vi "Station Detail Main.vi"(8 "error in (no error)":errorcluster, 11 "Vision AI in":refnum<class "Vision AI.lvclass">) -> (0 "error out":errorcluster, 2 "Station Out":T1=enum."ImformOut", 3 "Vision AI out":refnum<class "Vision AI.lvclass">)   [LabVIEW 2019, in "Vision AI.lvclass"]
uses:
  Vision AI.lvclass
  Ctrl/Station Action.ctl
  Ctl/VisionAI Act Step.ctl
  Ctl/S8 PLC to PC Output.ctl
  Ctrl/Auto Inspection Station Name2.ctl
  Ctrl/Auto Inspection Data Name.ctl
  Function/UpVision/Ctrl/UpColorImg.ctl
  <vilib>/userdefined/High Color/IMAQdx.ctl
  Ctl/S8 Station IO.ctl
  Ctrl/ModbusCmd.ctl
  Global/Process Global.vi
  LLB/Commonly VI/Main Glb.vi
  LLB/Commonly VI.lvlib
  Ctrl/MeasureDisplayTab.ctl
  Ctrl/Table Save.ctl
  <vilib>/vision/driver/NI_Vision_Acquisition_Software.lvlib
panel:
  out "CutPath":path[](array[path])
  out "body":string
  out "headers":string
  in  "站別":i32
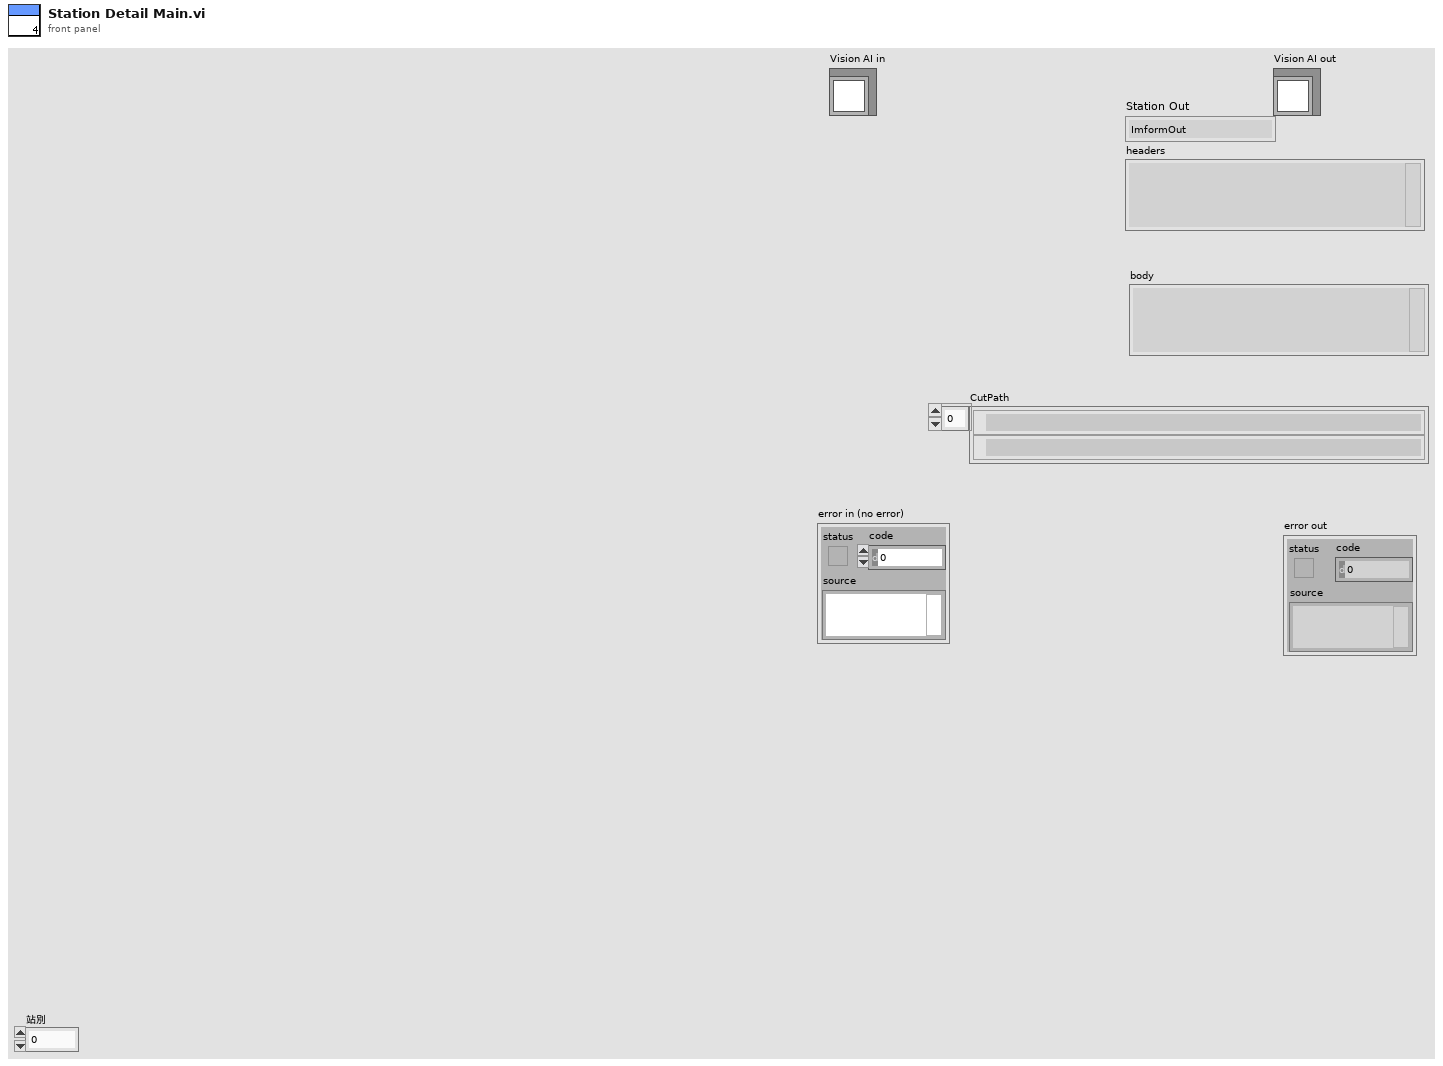
[diagram p1: front panel]
types:
  T1 = typedef "Station Action.ctl" = enum16{"Wait Item In", "Dectect Action", "ImformOut"}
  T2 = typedef "VisionAI Act Step.ctl" = enum16{"Initial", "VisionCheck1", "VisionGrab", "VisionSendToAI", "Vision1Finish", "VisionCheck2", "Vision2Finish", "DataCheck", "NGWay", "OKWay", "DataSave", "Finish"}
  T3 = typedef "S8 PLC to PC Output.ctl" = enum16{"S8 Vision AI載盤有料"}
  T4 = typedef "Auto Inspection Data Name.ctl" = enum16{"LocalRun", "ItemSN(TimeCode)", "CurrentAction", "Error", "Data", "OKNG", "電壓值", "電壓值判斷", "電流值", "電流值判斷", "Laser1 Data", "Laser2 Data", "Laser OKNG", "StationNO"}
  T5 = typedef "Auto Inspection Station Name2.ctl" = enum16{"S1Barcode", "S2Measure", "S3Measure", "S4Measure", "S5Measure", "S11_LaserCheck", "S8_Vision AI"}
  T6 = typedef "UpColorImg.ctl" = enum16{"CUpCam", "CUpSource", "CUpShow", "CUpToProcess1", "CUpToProcess2", "CUpForMatch", "CUpForCheckNumbers", "CupPreProcess"}
  T7 = typedef "IMAQdx.ctl" = refnum<k21>
  T8 = typedef "S8 Station IO.ctl" = enum16{"S8_PC動作中(address 80)", "S8 AI 浪代OK(address 81)", "S8 AI 浪代NG(address 82)", "S8 AI 動作完成"}
  T9 = cluster{"starting address":u16, "number of inputs":u16, "Sat Coils":bool[], "Holding Registers":u16[]}
  T10 = typedef "ModbusCmd.ctl" = enum16{"Connect", "Disconnect", "Init", "Fetch Basic Objects", "Fetch Input Refisters", "Fetch Discrete Inputs", "Set Coils", "Set Holding Registers", "Write Single Holding", "Exit"}
  T11 = typedef "MeasureDisplayTab.ctl" = enum16{"Tray Barcode", "PCBA BARCODE", "硬體(Tool初始化)", "company(Tool初始化)", "耗電流 uA(電流表)", "電池負載電壓", "晶片ID(Tool FORMAT)", "雷雕ID(TOOl scan、藍芽接收器)", "Format(Tool FORMAT)", "Programe(Tool Programe)", "MAC(藍芽接收器)", "ID(藍芽接收器)", "KPA(藍芽接收器)", "溫度(藍芽接收器)", "SENSOR電池電壓(藍芽接收器)", "RSSI(藍芽接收器)", "SensorType_315(FSK scan)", "FSKsnVol_315(FSK scan)", "FSKscanl_315(FSK scan)", "P_315(FSK scan)", "T_315(FSK scan)", "SensorType_433(ASK scan)", "ASKsnVol_433(ASK scan)", "ASKscan_433(ASK scan)", "P_433(ASK scan)", "T_433(ASK scan)", "測高Data"}
  T12 = typedef "Table Save.ctl" = enum16{"initial", "Add", "Write", "Replace", "Delete", "REad", "RedTable", "Load"}
  T13 = typedef "IMAQ Image.ctl" = refnum<image>
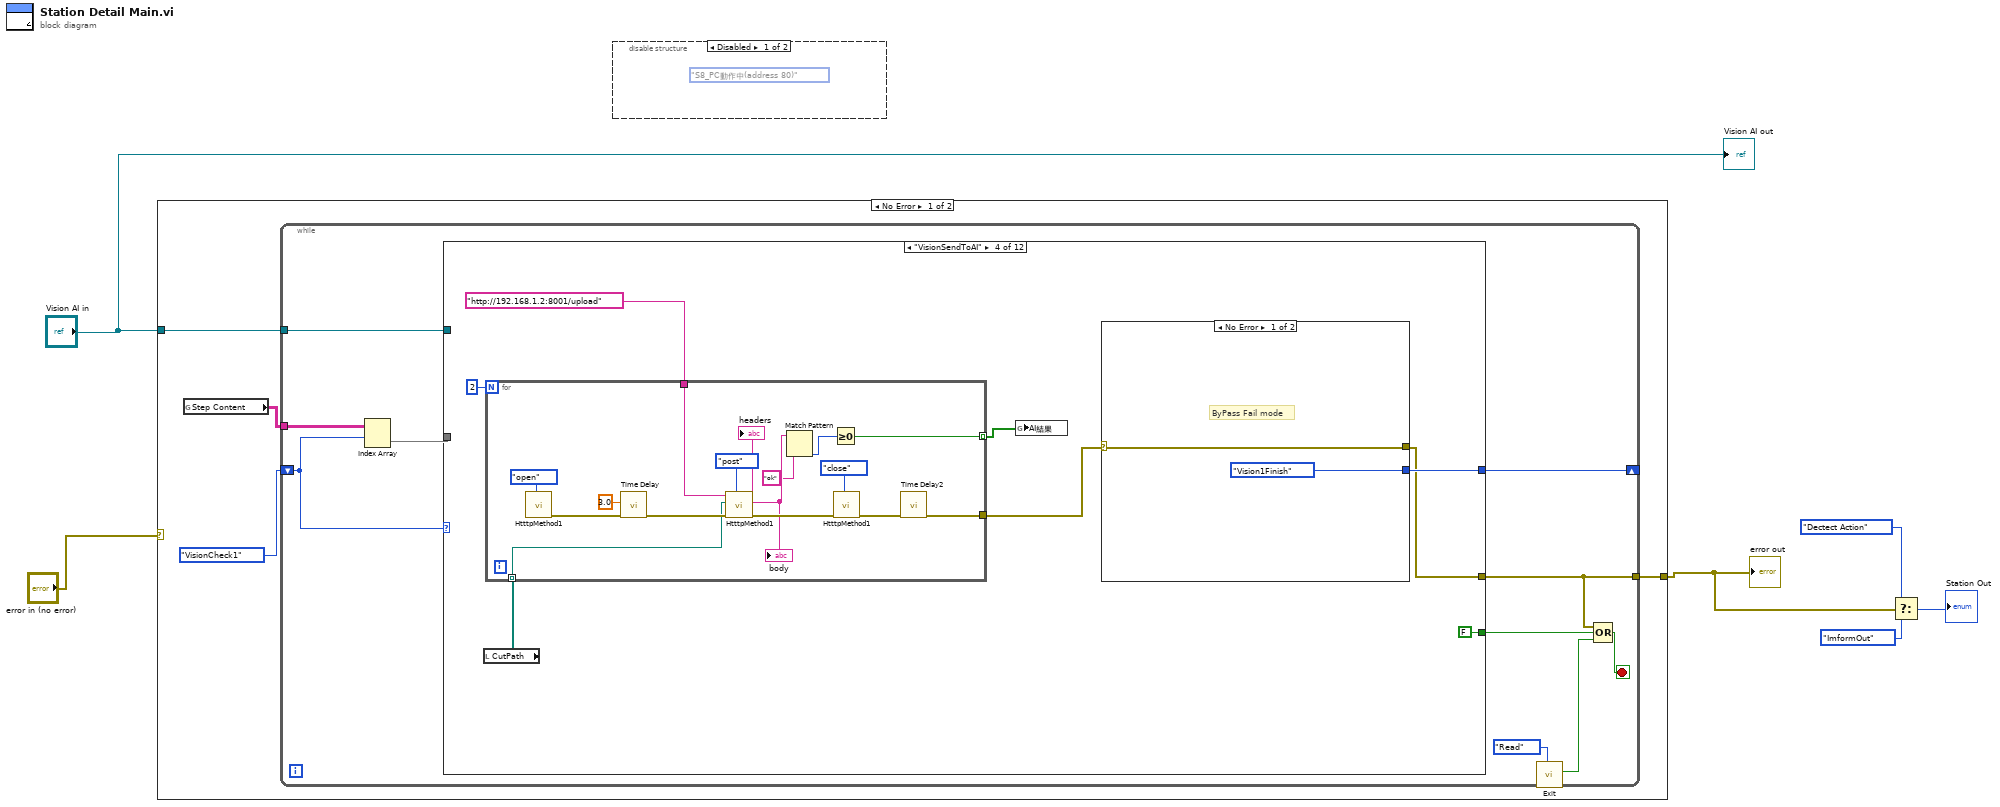
[diagram p0: block diagram]
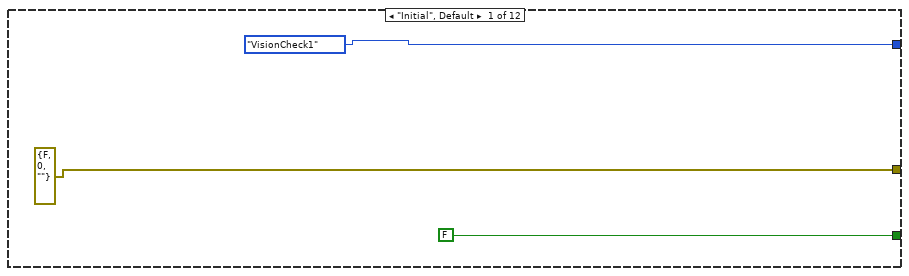
[diagram p3: hidden frame]
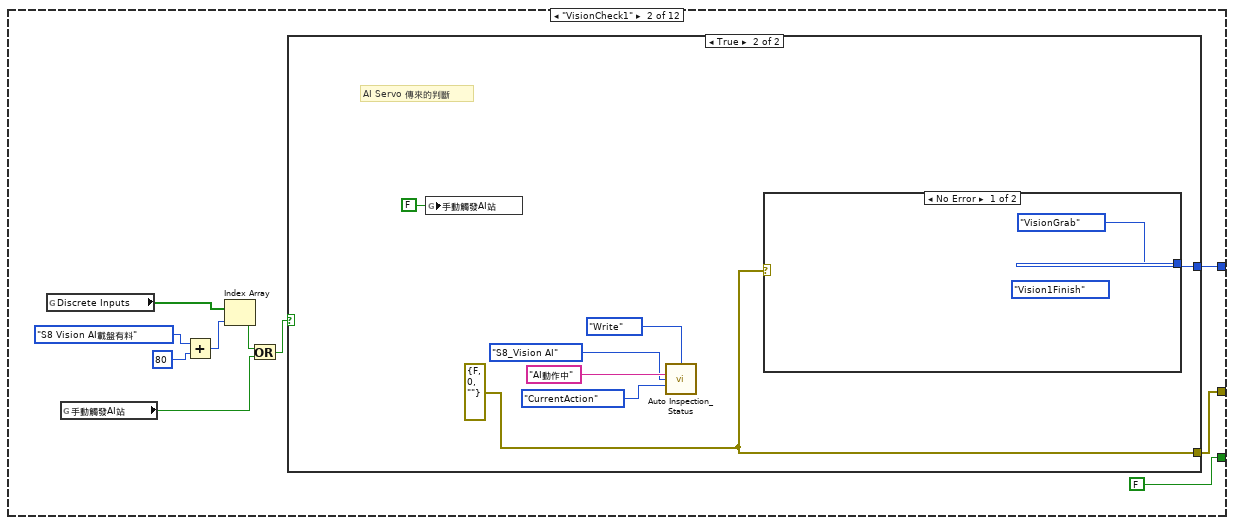
[diagram p4: hidden frame]
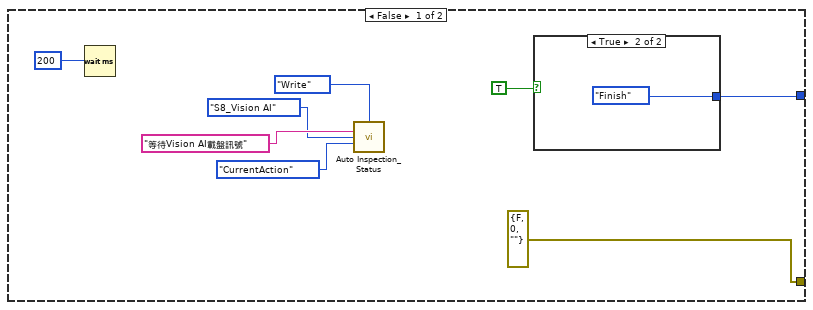
[diagram p5: hidden frame]
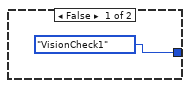
[diagram p6: hidden frame]
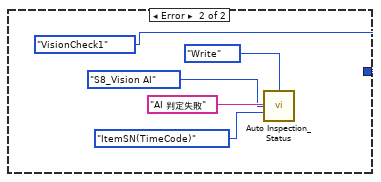
[diagram p7: hidden frame]
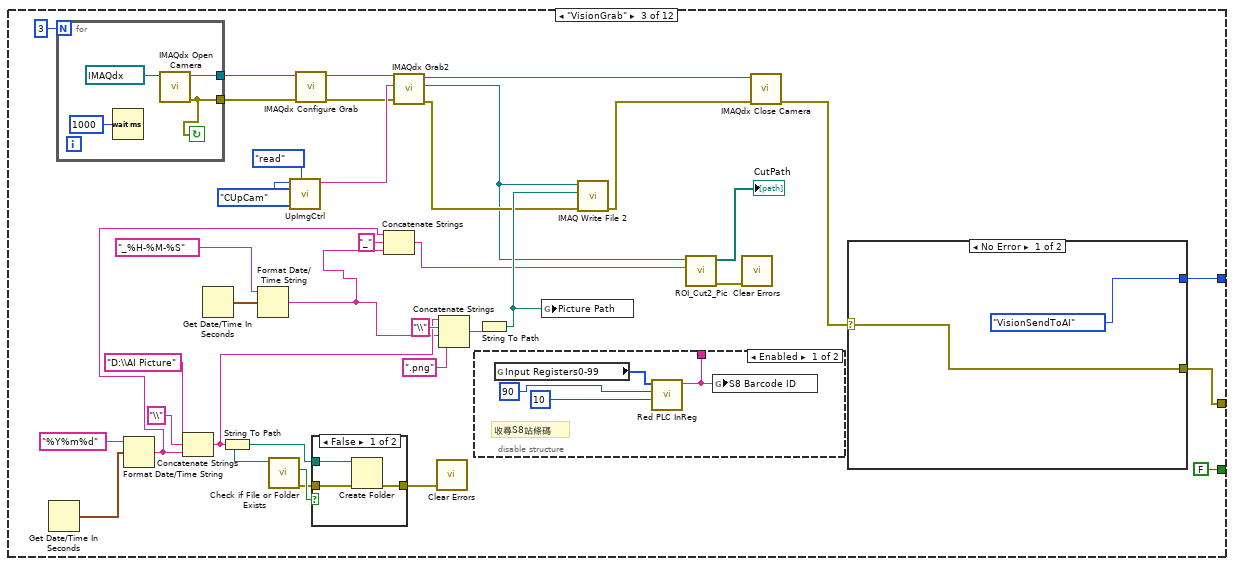
[diagram p8: hidden frame]
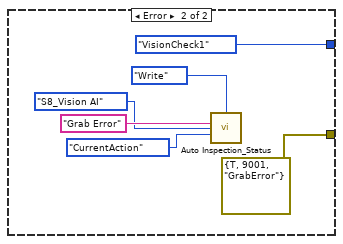
[diagram p11: hidden frame]
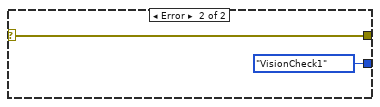
[diagram p12: hidden frame]
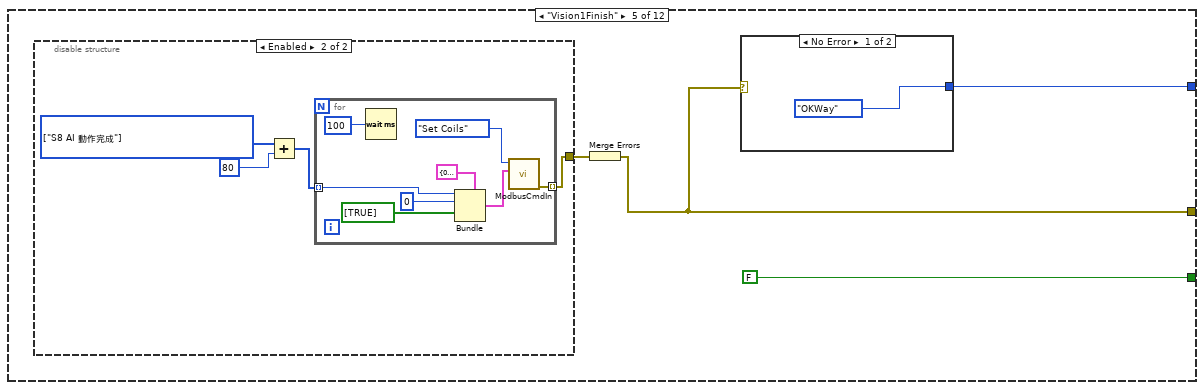
[diagram p13: hidden frame]
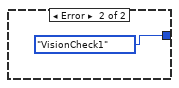
[diagram p14: hidden frame]
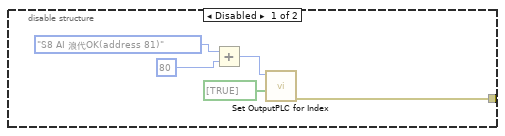
[diagram p15: hidden frame]
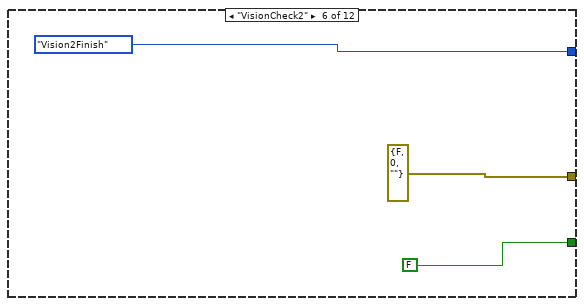
[diagram p16: hidden frame]
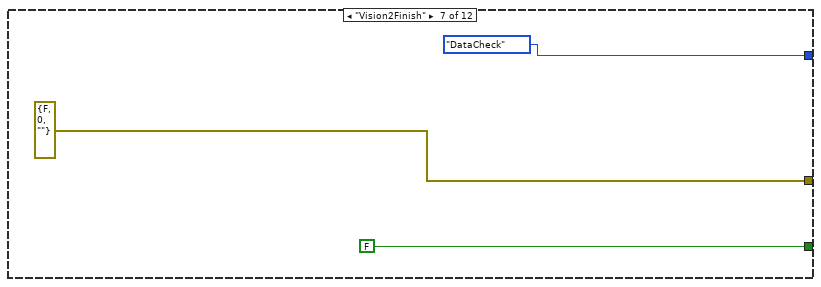
[diagram p17: hidden frame]
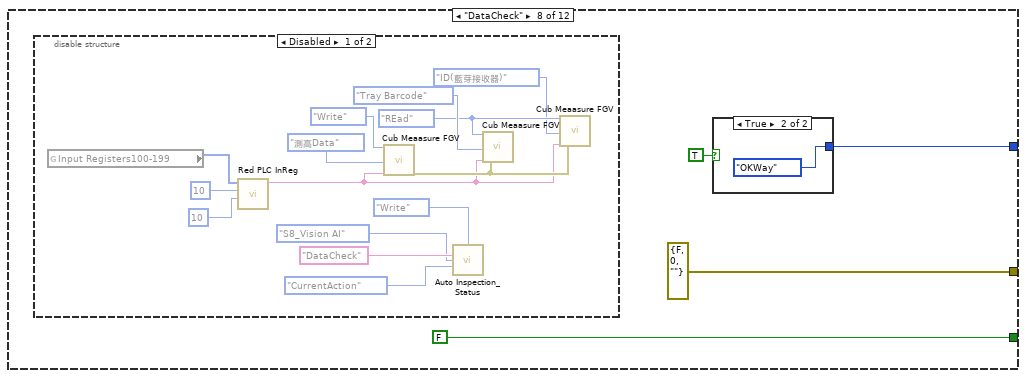
[diagram p18: hidden frame]
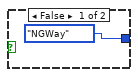
[diagram p20: hidden frame]
diagram:
  n1 = case shown="No Error" "error in (no error)" {
    selector: "error in (no error)" -> [_ w221]
    tunnel: [w10 w221] -> w2
    tunnel: "Vision AI in" -> [w8 _]
    frame No Error {
      n2 = global read "Process Global.vi" "Step Content"() -> (w9:string[][])
      n3 = while {
        tunnel: [w16] -> w10
        shift-right: [w20] -> _
        shift-left: VisionAI_Act_Step."VisionCheck1" ("Enum") -> [w17]
        tunnel: w9 -> [w18]
        tunnel: w8 -> [w11]
        stop <- w15 stop-if-true
        n4 = Index Array(array=w18, index (row)=w17) -> (element=w19:string[])  [unwired: 1 in]
        n5 = case shown="\"VisionSendToAI\"" w17 {
          tunnel: [errorcluster {"status"=FALSE, "code"=0, "source"=""} ("error constant") w31 w86 w118 w142 errorcluster {"status"=FALSE, "code"=0, "source"=""} ("error IO") errorcluster {"status"=FALSE, "code"=0, "source"=""} ("error IO") errorcluster {"status"=FALSE, "code"=0, "source"=""} ("error IO") w201 w213 errorcluster {"status"=FALSE, "code"=0, "source"=""} ("error IO") errorcluster {"status"=FALSE, "code"=0, "source"=""} ("error IO")] -> w16
          tunnel: [VisionAI_Act_Step."VisionCheck1" ("Enum") w33 w87 w121 w144 VisionAI_Act_Step."Vision2Finish" ("Enum") VisionAI_Act_Step."DataCheck" ("Enum") w174 VisionAI_Act_Step."Finish" ("Enum") VisionAI_Act_Step."DataSave" ("Enum") VisionAI_Act_Step."Finish" ("Enum") VisionAI_Act_Step."VisionCheck1" ("Enum")] -> w20
          tunnel: w19 -> [_ _ _ _ _ _ _ _ _ _ _ _]
          tunnel: [FALSE FALSE FALSE FALSE FALSE FALSE FALSE FALSE FALSE FALSE FALSE TRUE] -> w14
          tunnel: w11 -> [_ _ _ _ _ _ _ _ _ _ _ _]
          frame "Initial", Default {
          }
          frame "VisionCheck1" {
            n6 = global read "Main Glb.vi" "Discrete Inputs"() -> (w30:bool[])
            n7 = global read "Main Glb.vi" "手動觸發AI站"() -> (w24:bool)
            n8 = Add(x=S8_PLC_to_PC_Output."S8 Vision AI載盤有料" ("Enum"), y=80) -> (x+y=w29:i32)
            n9 = Index Array(array=w30, index=w29) -> (element=w26:bool)
            n10 = Or(x=w26, y=w24) -> (x .or. y?=w25:bool)
            n11 = case shown="True" w25 {
              tunnel: [w35 w50] -> w33
              tunnel: [errorcluster {"status"=FALSE, "code"=0, "source"=""} ("error out") w49] -> w31
              frame False {
                n12 = Wait (ms)(milliseconds to wait=200) -> ()  [unwired: 1 out]
                n13 = call "Auto Inspection_Status.vi"("Action"=enum16{"Initial", "Write", "Read"}."Write", "DataIn"="等待Vision AI載盤訊號", "Station"=Auto_Inspection_Station_Name2."S8_Vision AI", "Data"=Auto_Inspection_Data_Name."CurrentAction") -> ()  [unwired: 9 in, 3 out]
                n14 = case shown="True" TRUE {
                  tunnel: [VisionAI_Act_Step."VisionCheck1" ("Enum") VisionAI_Act_Step."Finish" ("Enum")] -> w35
                  frame False {
                  }
                  frame True {
                  }
                }
              }
              frame True {
                w49 = errorcluster {"status"=FALSE, "code"=0, "source"=""} ("error out")
                # "AI Servo 傳來的判斷"
                n15 = global write "Main Glb.vi" "手動觸發AI站"(FALSE ("手動觸發AI站")) -> ()
                n16 = call "Auto Inspection_Status.vi"("Action"=enum16{"Initial", "Write", "Read"}."Write", "DataIn"="AI動作中", "Station"=Auto_Inspection_Station_Name2."S8_Vision AI", "Data"=Auto_Inspection_Data_Name."CurrentAction") -> ()  [unwired: 9 in, 3 out]
                n17 = case shown="No Error" w49 {
                  tunnel: [VisionAI_Act_Step."VisionGrab" ("Enum") VisionAI_Act_Step."VisionCheck1" ("Enum")] -> w50
                  frame No Error {
                    (unwired) VisionAI_Act_Step."Vision1Finish" ("Enum")
                  }
                  frame Error {
                    n18 = call "Auto Inspection_Status.vi"("Action"=enum16{"Initial", "Write", "Read"}."Write", "DataIn"="AI 判定失敗", "Station"=Auto_Inspection_Station_Name2."S8_Vision AI", "Data"=Auto_Inspection_Data_Name."ItemSN(TimeCode)") -> ()  [unwired: 9 in, 3 out]
                  }
                }
              }
            }
          }
          frame "VisionGrab" {
            n19 = Get Date/Time In Seconds() -> (seconds since 1Jan1904=w62:timestamp)
            n20 = for {
              N: 3 -> [_]
              tunnel: [w100] -> w67
              tunnel: [w99] -> w66
              stop <- w100 continue-if-true
              n21 = Wait (ms)(milliseconds to wait=u32 1000) -> ()  [unwired: 1 out]
              n22 = call <vilib>:"IMAQdx Open Camera.vi"("Session In"=T7 "cam0") -> ("error out"=w100:errorcluster, "Session Out"=w99:T7)  [unwired: 9 in]
            }
            n23 = Format Date/Time String(time format string (%c)="%Y%m%d", seconds (now)=w62) -> (date/time string=w58:string)  [unwired: 1 out]
            n24 = Concatenate Strings("D:\\AI Picture" ("string"), "\\" ("string"), w58) -> (w73:string)
            n25 = Get Date/Time In Seconds() -> (seconds since 1Jan1904=w79:timestamp)
            n26 = String To Path(string=w73) -> (path=w80:path)
            n27 = Format Date/Time String(time format string (%c)="_%H-%M-%S", seconds (now)=w79) -> (date/time string=w60:string)  [unwired: 1 in]
            n28 = call <vilib>:"Check if File or Folder Exists.vi"("path"=w80) -> ("error out"=w81:errorcluster, "file or folder exists?"=w82:bool)  [unwired: 1 in, 8 out]
            n29 = call "UpImgCtrl.vi"("Action"=enum16{"Initial", "read", "release"}."read", "ColorImg 2"=UpColorImg."CUpCam") -> ("ColorImg"=w89:string)  [unwired: 7 in, 2 out]
            n30 = call <vilib>:"IMAQdx Configure Grab.vi"("error in"=w67, "Session In"=w66) -> ("error out"=w70:errorcluster, "Session Out"=w69:T7)  [unwired: 8 in]
            n31 = case shown="False" w82 {
              tunnel: w80 -> [w104 _]
              tunnel: w81 -> [w103 w105]
              tunnel: [w102 w105] -> w78
              frame False {
                n32 = Create Folder(path (use dialog)=w104, error in=w103) -> (error out=w102:errorcluster)  [unwired: 3 out]
              }
              frame True {
              }
            }
            n33 = Concatenate Strings(w58, "_" ("string"), w60) -> (w57:string)
            n34 = call <vilib>:"IMAQdx Grab2.vi"("error in"=w70, "Image In"=w89, "Session In"=w69) -> ("error out"=w71:errorcluster, "Image Out"=w65:T13, "Session Out"=w91:T7)  [unwired: 5 in, 1 out]
            n35 = call <vilib>:"Clear Errors.vi"("error in (no error)"=w78) -> ()  [unwired: 5 in, 2 out]
            n36 = Concatenate Strings(w73, "\\" ("string"), w60, ".png" ("string")) -> (w75:string)
            n37 = disable-structure shown="Enabled" {
              disable-tunnel: [w94 _] -> _
              frame Enabled {
                # "收尋S8站條碼"
                n38 = global read "Main Glb.vi" "Input Registers0-99"() -> (w97:u16[])
                n39 = call "Red PLC InReg.vi"("length"=10, "index"=90, "Input Registers Arr"=w97) -> ("Rad In Reg"=w94:string)  [unwired: 7 in, 1 out]
                n40 = global write "Main Glb.vi" "S8 Barcode ID"(w94) -> ()
              }
              frame Disabled {
              }
            }
            n41 = String To Path(string=w75) -> (path=w72:path)
            n42 = global write "Main Glb.vi" "Picture Path"(w72) -> ()
            n43 = call-poly "IMAQ Write File 2"("error in (no error)"=w71, "File Path"=w72, "Image"=w65) -> ("error out"=w77:errorcluster)  [unwired: 7 in, 1 out]
            n44 = call "ROI_Cut2_Pic.vi"("Name"=w57, "Image Org In"=w65) -> ("error out"=w64:errorcluster, "CutPath"=→"CutPath":path[])  [unwired: 8 in]
            n45 = call <vilib>:"Clear Errors.vi"("error in (no error)"=w64) -> ()  [unwired: 5 in, 2 out]
            n46 = call <vilib>:"IMAQdx Close Camera.vi"("error in"=w77, "Session In"=w91) -> ("error out"=w88:errorcluster)  [unwired: 9 in]
            n47 = case shown="No Error" w88 {
              selector: w88 -> [w106 _]
              tunnel: [VisionAI_Act_Step."VisionSendToAI" ("Enum") VisionAI_Act_Step."VisionCheck1" ("Enum")] -> w87
              tunnel: [w106 errorcluster {"status"=TRUE, "code"=9001, "source"="GrabError"} ("error IO")] -> w86
              frame No Error {
              }
              frame Error {
                n48 = call "Auto Inspection_Status.vi"("Action"=enum16{"Initial", "Write", "Read"}."Write", "DataIn"="Grab Error", "Station"=Auto_Inspection_Station_Name2."S8_Vision AI", "Data"=Auto_Inspection_Data_Name."CurrentAction") -> ()  [unwired: 9 in, 3 out]
              }
            }
          }
          frame "VisionSendToAI" {
            n49 = local read "CutPath"() -> (w115:path[])
            n50 = for {
              N: 2 -> [_]
              tunnel: "http://192.168.1.2:8001/upload" ("url") -> [w136]
              tunnel: [w125] -> w117
              tunnel: [w124] -> w116 mode=indexing
              tunnel: w115 -> [w122] mode=indexing
              n51 = call "HtttpMethod1.vi"("http"=enum16{"open", "post", "close", "idle"}."open") -> ("error out"=w132:errorcluster)  [unwired: 8 in, 2 out]
              n52 = call "Time Delay"("error in (no error)"=w132, "Delay Time (s)"=3.0) -> ("error out"=w131:errorcluster)  [unwired: 9 in]
              n53 = call "HtttpMethod1.vi"("http"=enum16{"open", "post", "close", "idle"}."post", "error constant"=w131, "file"=w122, "url"=w136) -> ("error out"=w133:errorcluster, "body"=w127:string, "headers"=→"headers":string)  [unwired: 5 in]
              "body" <- w127
              n54 = Match Pattern(string=w127, regular expression="ok") -> (offset past match=w126:i32)  [unwired: 1 in, 3 out]
              n55 = Greater Or Equal To 0?(x=w126) -> (x >= 0?=w124:bool)
              n56 = call "HtttpMethod1.vi"("http"=enum16{"open", "post", "close", "idle"}."close", "error constant"=w133) -> ("error out"=w129:errorcluster)  [unwired: 7 in, 2 out]
              n57 = call "Time Delay2"("error in (no error)"=w129) -> ("error out"=w125:errorcluster)  [unwired: 10 in]
            }
            n58 = global write "Process Global.vi" "AI結果"(w116) -> ()
            n59 = case shown="No Error" w117 {
              selector: w117 -> [w138 w140]
              tunnel: [VisionAI_Act_Step."Vision1Finish" ("Enum") VisionAI_Act_Step."VisionCheck1" ("Enum")] -> w121
              tunnel: [w138 w140] -> w118
              frame No Error {
                # "ByPass Fail mode"
              }
              frame Error {
              }
            }
          }
          frame "Vision1Finish" {
            n60 = disable-structure shown="Enabled" {
              disable-tunnel: [w152 w153] -> w145
              frame Disabled {
                n61 = Add(x=S8_Station_IO."S8 AI 浪代OK(address 81)" ("Enum"), y=80) -> (x+y=w149:i32)
                n62 = call "Set OutputPLC for Index.vi"("Index"=w149, "Sat Coils"=bool[] [TRUE]) -> ("Error Out"=w152:errorcluster[])  [unwired: 8 in]
              }
              frame Enabled {
                w154 = T8[] [enum."S8 AI 動作完成"] items=["S8_PC動作中(address 80)", "S8 AI 浪代OK(address 81)", "S8 AI 浪代NG(address 82)", "S8 AI 動作完成"]
                n63 = Add(x=w154, y=80) -> (x+y=w156:i32[])
                n64 = for {
                  tunnel: [w158] -> w153 mode=indexing
                  tunnel: w156 -> [w157] mode=indexing
                  n65 = Wait (ms)(milliseconds to wait=100) -> ()  [unwired: 1 out]
                  n66 = Bundle(cluster=T9 {"starting address"=0, "number of inputs"=0, "Sat Coils"=[], "Holding Registers"=[]} ("data"), "starting address"=w157, "number of inputs"=u16 0, "Sat Coils"=bool[] [TRUE]) -> (w161:T9)  [unwired: 1 in]
                  n67 = call "ModbusCmdIn.vi"("data"=w161, "Enum"=ModbusCmd."Set Coils") -> ("error out"=w158:errorcluster)  [unwired: 9 in]
                }
              }
            }
            n68 = Merge Errors(w145) -> (w142:errorcluster)
            n69 = case shown="No Error" w142 {
              tunnel: [VisionAI_Act_Step."OKWay" ("Enum") VisionAI_Act_Step."VisionCheck1" ("Enum")] -> w144
              frame No Error {
              }
              frame Error {
              }
            }
          }
          frame "VisionCheck2" {
          }
          frame "Vision2Finish" {
          }
          frame "DataCheck" {
            n70 = disable-structure shown="Disabled" {
              frame Disabled {
                w178 = Table_Save."REad" ("Enum")
                n71 = global read "Main Glb.vi" "Input Registers100-199"() -> (w180:u16[])
                n72 = call "Red PLC InReg.vi"("length"=10, "index"=10, "Input Registers Arr"=w180) -> ("Rad In Reg"=w176:string)  [unwired: 7 in, 1 out]
                n73 = call "Cub Meaasure FGV.vi"("Action"=Table_Save."Write" ("Enum"), "Save Index"=MeasureDisplayTab."測高Data", "SN"=w176) -> ("error out"=w177:errorcluster)  [unwired: 9 in, 7 out]
                n74 = call "Auto Inspection_Status.vi"("Action"=enum16{"Initial", "Write", "Read"}."Write", "DataIn"="DataCheck", "Station"=Auto_Inspection_Station_Name2."S8_Vision AI", "Data"=Auto_Inspection_Data_Name."CurrentAction") -> ()  [unwired: 9 in, 3 out]
                n75 = call "Cub Meaasure FGV.vi"("Action"=w178, "Save Index"=MeasureDisplayTab."Tray Barcode", "SN"=w176, "error in (no error)"=w177) -> ()  [unwired: 8 in, 8 out]
                n76 = call "Cub Meaasure FGV.vi"("Action"=w178, "Save Index"=MeasureDisplayTab."ID(藍芽接收器)", "SN"=w176, "error in (no error)"=w177) -> ()  [unwired: 8 in, 8 out]
              }
              frame Enabled {
              }
            }
            n77 = case shown="True" TRUE {
              tunnel: [VisionAI_Act_Step."NGWay" ("Enum") VisionAI_Act_Step."OKWay" ("Enum")] -> w174
              frame False {
              }
              frame True {
              }
            }
          }
          frame "NGWay" {
            n78 = Add(x=S8_Station_IO."S8 AI 浪代NG(address 82)" ("Enum"), y=80) -> (x+y=w193:i32)
            n79 = call "Auto Inspection_Status.vi"("Action"=enum16{"Initial", "Write", "Read"}."Write", "DataIn"="AI判斷 NG", "Station"=Auto_Inspection_Station_Name2."S8_Vision AI", "Data"=Auto_Inspection_Data_Name."OKNG") -> ()  [unwired: 9 in, 3 out]
            n80 = call "Set OutputPLC for Index.vi"("Index"=w193, "Sat Coils"=bool[] [TRUE]) -> ("Error Out"=w191:errorcluster[])  [unwired: 8 in]
            n81 = Merge Errors(w191) -> (w201:errorcluster)
          }
          frame "OKWay" {
            # "給PLC訊號"
            n82 = call "Auto Inspection_Status.vi"("Action"=enum16{"Initial", "Write", "Read"}."Write", "DataIn"="AI判斷 OK", "Station"=Auto_Inspection_Station_Name2."S8_Vision AI", "Data"=Auto_Inspection_Data_Name."OKNG") -> ()  [unwired: 9 in, 3 out]
            n83 = Add(x=S8_Station_IO."S8 AI 浪代OK(address 81)" ("Enum"), y=80) -> (x+y=w206:i32)
            n84 = call "Set OutputPLC for Index.vi"("Index"=w206, "Sat Coils"=bool[] [TRUE]) -> ("Error Out"=w203:errorcluster[])  [unwired: 8 in]
            n85 = Merge Errors(w203) -> (w213:errorcluster)
          }
          frame "DataSave" {
          }
          frame "Finish" {
          }
        }
        n86 = call "Exit.vi"("Enum"=enum16{"Initial", "Read", "Write"}."Read") -> ("ExitOut"=w12:bool)  [unwired: 10 in]
        n87 = Compound Arithmetic op=OR(w16, w14, w12) -> (w15:bool)
      }
    }
    frame Error {
    }
  }
  "error out" <- w2
  n88 = disable-structure shown="Disabled" {
    frame Disabled {
      (unwired) S8_Station_IO."S8_PC動作中(address 80)" ("Enum")
    }
    frame Enabled {
    }
  }
  n89 = Select(t=Station_Action."Dectect Action" ("Station Out"), s=w2, f=Station_Action."ImformOut" ("Station Out")) -> (s? t:f=→"Station Out":T1)
  "Vision AI out" <- "Vision AI in"
